vi "set_run_mode.vi"(8 "error in (no error)":errorcluster, 10 "run mode":T1=enum."single sweep mode", 11 "GenericPlugin in":refnum<class "GenericComponent.lvclass">) -> (0 "error out":errorcluster, 3 "GenericPlugin out":refnum<class "GenericComponent.lvclass">)   [LabVIEW 2010, in "GenericComponent.lvclass"]
uses:
  GenericComponent.lvclass
  main/labview_source/type_definitions/enumerations/run_mode_enum.ctl
  components/ExperimentController/GenericExperimentController/GenericExperimentController/trigger_enum.ctl
  components/ExperimentController/GenericExperimentController/GenericExperimentController/GenericExperimentController.lvclass
  components/DAQ/GenericDAQ/GenericDAQ/GenericDAQ.lvclass
  components/ScanHead/GenericScanHead/GenericScanHead/GenericScanHead.lvclass
  components/ScanHead/GenericScanHead/GenericScanHead/trigger_enum.ctl
  class_data.vi
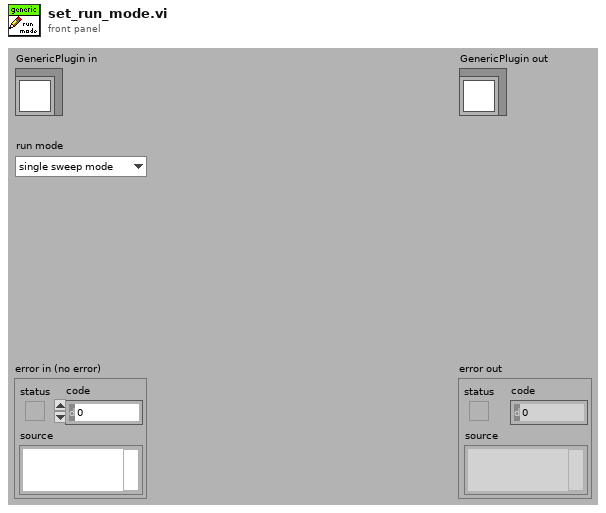
[diagram p1: front panel]
types:
  T1 = typedef "run_mode_enum.ctl" = enum16{"focus mode", "single sweep mode", "experiment mode"}
  T2 = typedef "GenericExperimentController.lvclass/trigger_enum.ctl" = enum16{"NULL", "proceed", "prepare"}
  T3 = typedef "GenericScanHead.lvclass/trigger_enum.ctl" = enum16{"NULL", "fetch trajectory", "generate trajectory", "change run mode", "update modifiers"}
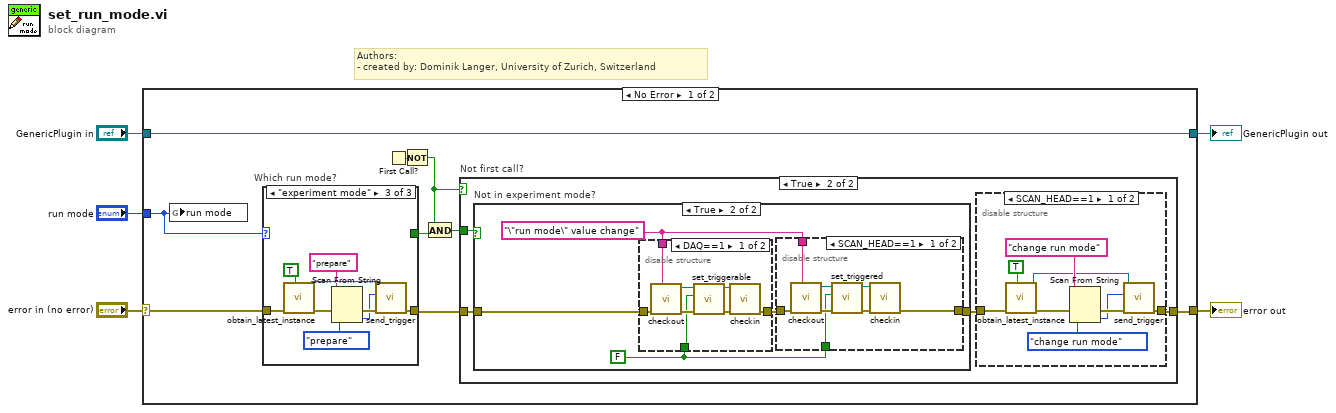
[diagram p0: block diagram]
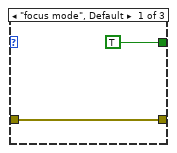
[diagram p2: hidden frame]
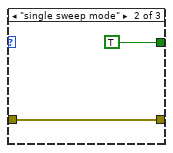
[diagram p3: hidden frame]
diagram:
  # "Authors: \n- created by: Dominik Langer, University of Zurich, Switzerland"
  n1 = case shown="No Error" "error in (no error)" {
    selector: "error in (no error)" -> [w12 w68]
    tunnel: [w13 w68] -> w4
    tunnel: [w14 w67] -> w2
    tunnel: "GenericPlugin in" -> [w14 w67]
    tunnel: "run mode" -> [w10 _]
    frame No Error {
      n2 = global write "class_data.vi" "run mode"(w10) -> ()
      n3 = case "Which run mode?" shown="\"experiment mode\"" w10 {
        tunnel: [TRUE TRUE _] -> w9
        tunnel: w12 -> [w15 w17 w21]
        tunnel: [w15 w17 w25] -> w11
        frame "focus mode", Default {
        }
        frame "single sweep mode" {
        }
        frame "experiment mode" {
          n4 = call "obtain_latest_instance.vi"("quick, but maybe outdated?"=TRUE, "error in (no error)"=w21) -> ("error out"=w24:errorcluster, "GenericExperimentController out"=w27:refnum<class "GenericExperimentController.lvclass">)  [unwired: 8 in]
          n5 = Scan From String(input string="prepare", error in=w24, default 1=trigger_enum."prepare" ("trigger")) -> (error out=w22:errorcluster, output 1=w20:T2)  [unwired: 2 in, 2 out]
          n6 = call-dynamic "send_trigger.vi"("error in (no error)"=w22, "trigger"=w20, "GenericExperiment in"=w27) -> ("error out"=w25:errorcluster)  [unwired: 7 in, 1 out]
        }
      }
      n7 = First Call?() -> (First Call?: T/F=w7:bool)
      n8 = Not(x=w7) -> (.not. x?=w6:bool)
      n9 = And(x=w6, y=w9) -> (x .and. y?=w8:bool)
      n10 = case "Not first call?" shown="True" w6 {
        tunnel: w11 -> [w28 w31]
        tunnel: [w28 w32] -> w13
        tunnel: w8 -> [_ w29]
        frame False {
        }
        frame True {
          n11 = case "Not in experiment mode?" shown="True" w29 {
            tunnel: w31 -> [w43 w48]
            tunnel: [w43 w46] -> w30
            frame False {
            }
            frame True {
              w45 = FALSE ("triggerable?")
              w44 = "\"run mode\" value change" ("locked by?")
              n12 = disable-structure shown="DAQ==1" {
                disable-tunnel: w48 -> [w52 w57]
                disable-tunnel: [w51 w57] -> w47
                disable-tunnel: w45 -> [w50 _]
                disable-tunnel: w44 -> [w49 _]
                frame condition #0 (active) {
                  n13 = call "checkout.vi"("locked by?"=w49, "error in (no error)"=w52) -> ("error out"=w56:errorcluster, "GenericDAQ out"=w54:refnum<class "GenericDAQ.lvclass">)  [unwired: 8 out]
                  n14 = call-dynamic "set_triggerable.vi"("error in (no error)"=w56, "triggerable?"=w50, "GenericDAQ in"=w54) -> ("error out"=w55:errorcluster, "GenericDAQ out"=w53:refnum<class "GenericDAQ.lvclass">)  [unwired: 7 out]
                  n15 = call-dynamic "checkin.vi"("error in (no error)"=w55, "GenericDAQ in"=w53) -> ("error out"=w51:errorcluster)  [unwired: 8 in, 1 out]
                }
                frame condition #1 {
                }
              }
              n16 = disable-structure shown="SCAN_HEAD==1" {
                disable-tunnel: w47 -> [w61 w66]
                disable-tunnel: [w60 w66] -> w46
                disable-tunnel: w45 -> [w59 _]
                disable-tunnel: w44 -> [w58 _]
                frame condition #0 (active) {
                  n17 = call "checkout.vi"("locked by?"=w58, "error in (no error)"=w61) -> ("error out"=w63:errorcluster, "GenericScanHead out"=w64:refnum<class "GenericScanHead.lvclass">)  [unwired: 8 out]
                  n18 = call-dynamic "set_triggered.vi"("error in (no error)"=w63, "triggered?"=w59, "GenericScanHead.lvclass in"=w64) -> ("error out"=w62:errorcluster, "GenericScanHead.lvclass out"=w65:refnum<class "GenericScanHead.lvclass">)  [unwired: 7 out]
                  n19 = call-dynamic "checkin.vi"("error in (no error)"=w62, "GenericScanHead in"=w65) -> ("error out"=w60:errorcluster)  [unwired: 8 in, 1 out]
                }
                frame condition #1 {
                }
              }
            }
          }
          n20 = disable-structure shown="SCAN_HEAD==1" {
            disable-tunnel: [w40 w42] -> w32
            disable-tunnel: w30 -> [w39 w42]
            frame condition #0 (active) {
              n21 = call "obtain_latest_instance.vi"("quick, but maybe outdated?"=TRUE, "error in (no error)"=w39) -> ("error out"=w36:errorcluster, "GenericScanHead out"=w34:refnum<class "GenericScanHead.lvclass">)  [unwired: 8 out]
              n22 = Scan From String(input string="change run mode", error in=w36, default 1=trigger_enum."change run mode" ("trigger")) -> (error out=w35:errorcluster, output 1=w33:T3)  [unwired: 2 in, 2 out]
              n23 = call-dynamic "send_trigger.vi"("error in (no error)"=w35, "trigger"=w33, "GenericScanHead in"=w34) -> ("error out"=w40:errorcluster)  [unwired: 8 out]
            }
            frame condition #1 {
            }
          }
        }
      }
    }
    frame Error {
    }
  }
  "error out" <- w4
  "GenericPlugin out" <- w2
